vi "dequeue.vi"(8 "error in (no error)":errorcluster, 11 "comic_crawler.lvclass":refnum<class "comic_crawler.lvclass">) -> (0 "error out":errorcluster, 1 "data":variant, 2 "cmd":T1, 3 "comic_crawler.lvclass out":refnum<class "comic_crawler.lvclass">)   [LabVIEW 2024, in "comic_crawler.lvclass"]
uses:
  comic_crawler.lvclass
  comic_crawler.lvclass/comic_crawler.ctl
  daemon.states--enum.ctl
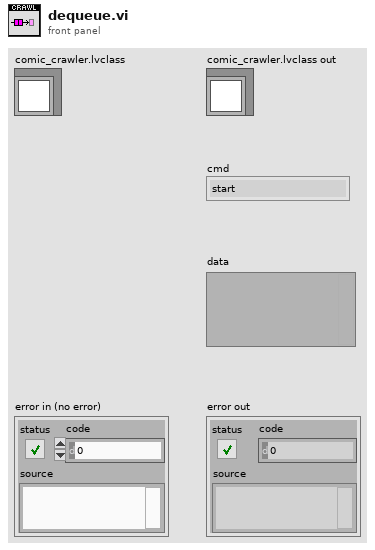
[diagram p1: front panel]
types:
  T1 = typedef "comic_crawler.lvclass/daemon.states--enum.ctl" = enum16{"start", "pause", "stop", "shut down"}
  T2 = typedef "comic_crawler.lvclass/queue.message--cluster.ctl" = cluster{"cmd":T1, "data":variant}
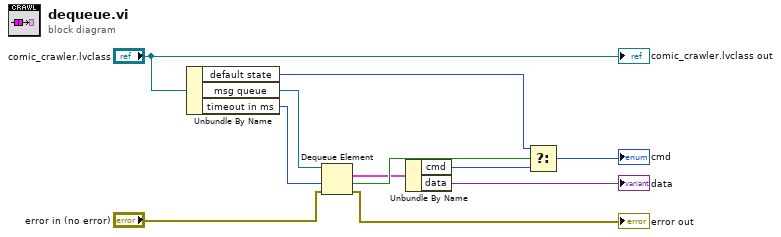
[diagram p0: block diagram]
diagram:
  n1 = Unbundle By Name("comic_crawler.lvclass") -> ("default state"=w3:T1, "msg queue"=w9:refnum<queue>, "timeout in ms"=w10:i32)
  n2 = Dequeue Element(queue=w9, timeout in ms (-1)=w10, error in (no error)="error in (no error)") -> (element=w5:T2, timed out?=w6:bool, error out=→"error out":errorcluster)  [unwired: 1 out]
  n3 = Unbundle By Name(w5) -> ("cmd"=w4:T1, "data"=→"data":variant)
  n4 = Select(t=w3, s=w6, f=w4) -> (s? t:f=→"cmd":T1)
  "comic_crawler.lvclass out" <- "comic_crawler.lvclass"
